vi "save_and_process_continious_image_data.vi"(0 "queue out":refnum<queue>, 1 "HDFvsTDMS":bool, 2 "Enable online recon":bool, 3 "Save":bool, 4 "Path for TDMS":path=path "C:/Users/MPI/Desktop", 5 "Subject metadata cluster":T2, 6 "Path":path=path "C:/Users/MPI/Desktop", 7 "System Information cluster":T1, 10 "OnlineReconPath":path) -> ()   [LabVIEW 2021]
uses:
  Human_Labview/global_variables.vi
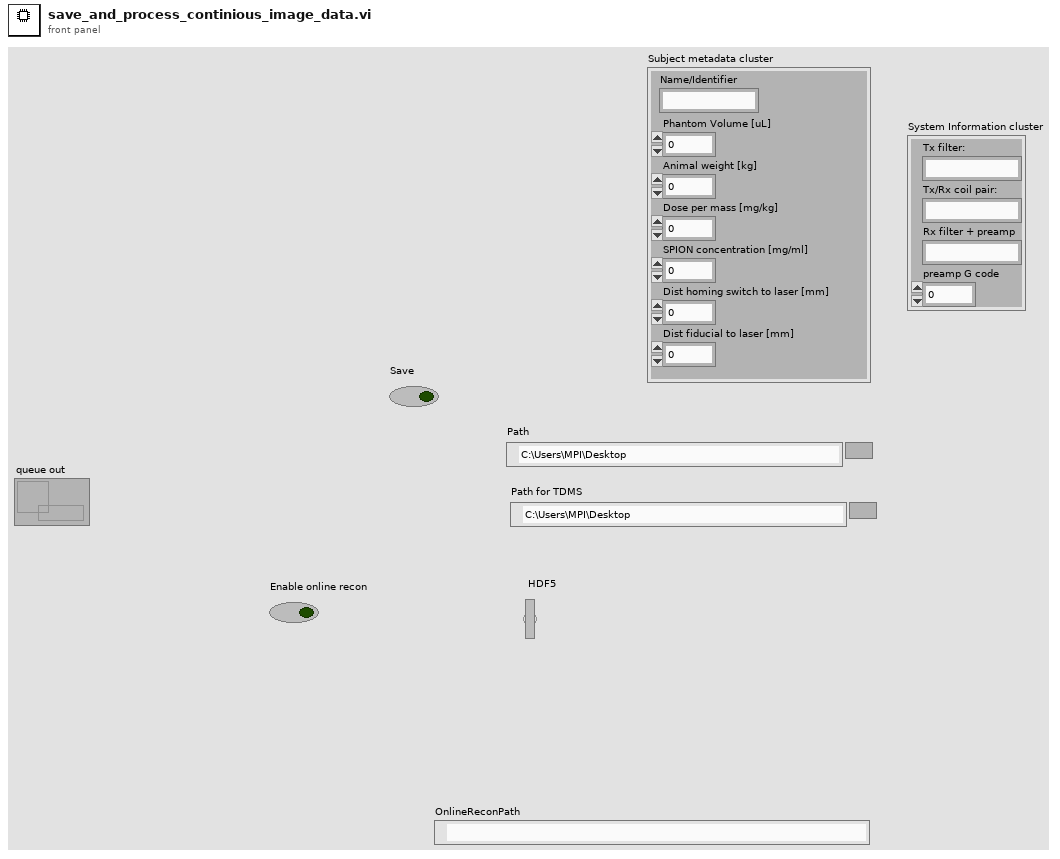
[diagram p1: front panel]
types:
  T1 = cluster{"Tx filter:":string, "Tx/Rx coil pair:":string, "Rx filter + preamp":string, "preamp G code":dbl}
  T2 = cluster{"Name/Identifier":string, "Phantom Volume [uL]":dbl, "Animal weight [kg]":dbl, "Dose per mass [mg/kg]":dbl, "SPION concentration [mg/ml]":dbl, "Dist homing switch to laser [mm]":dbl, "Dist fiducial to laser [mm]":dbl}
  T3 = cluster{"sample rate":dbl, "Transmit frequency":dbl, "Transmit amplitude":dbl, "sample rate digital out":dbl, "TX cycles":i32, "sample rate DAQ1":dbl, "Receive frequency":dbl, "Receive range":dbl, "TX harmonics":dbl[]}
  T4 = cluster{"Magnitude meas.":dbl[], "Phase meas.":dbl[], "Shift meas.":dbl[], "cw":bool, "projections per image":i32, "ramp-up readouts":i32, "current sense type":string, "Number of pulses per image":i32, "Rotation enabled":bool, "Rotary position":dbl[], "Baseline magnitude":dbl, "Baseline phase":dbl, "Wait readouts":i32, "Shift waveform type":string, "Shift enabled":bool, "Time domain data":dbl[], "Motor pulse duration":dbl, "Shift start":dbl, "Shift stop":dbl, "Notes":string, "Reconstructed image":picture, "Rotary encoder type":string, "Image start":timestamp, "Image stop":timestamp, "readouts per projection":i32, "Recon enabled":bool, "Bidirectional shift":bool, "Imager mode":string, "Shift delay":dbl, "Shift frequency":dbl, "Image time (calc)":dbl, "Initial encoder position":dbl, "Recon data":dbl[][], "Trigger line values":i32[], "Bed position":dbl, "Sample image":picture, "Patch amplitude":dbl, "Patch frequency":dbl, "Patch phase":dbl, "proj mag f2-f9":dbl[][], "proj phase f2-f9":dbl[][], "Tx waveform":dbl[], "Tx FFT mag":dbl[], "Tx FFT phase":dbl[], "Temps":dbl[]}
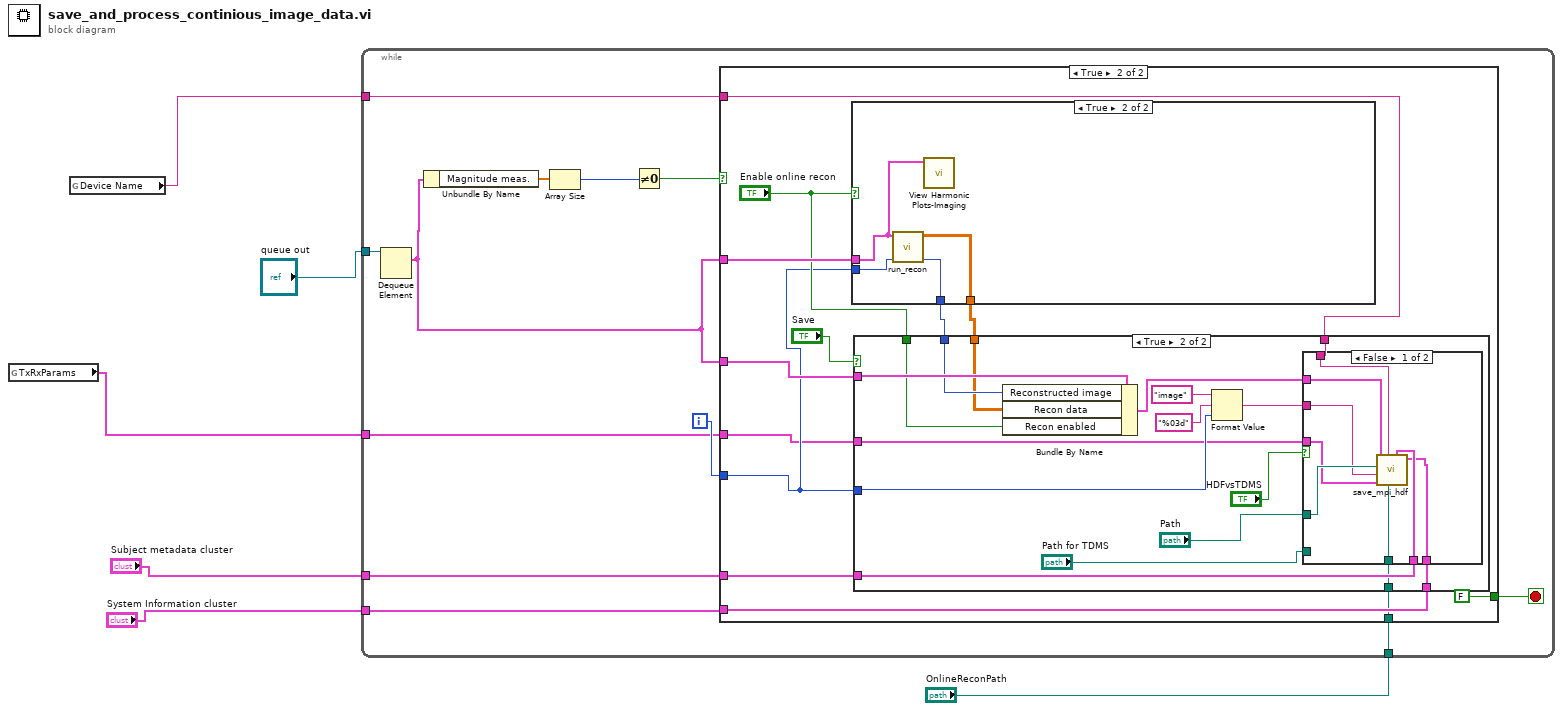
[diagram p0: block diagram]
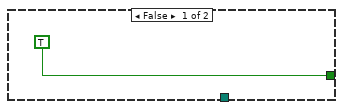
[diagram p2: hidden frame]
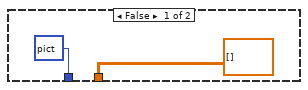
[diagram p3: hidden frame]
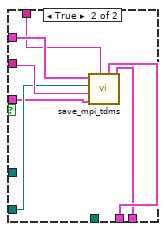
[diagram p5: hidden frame]
diagram:
  n1 = global read "global_variables.vi" "TxRxParams"() -> (w5:T3)
  n2 = global read "global_variables.vi" "Device Name"() -> (w4:tag)
  n3 = while {
    tunnel: "queue out" -> [w15]
    tunnel: w5 -> [w11]
    tunnel: w4 -> [w10]
    tunnel: "Subject metadata cluster" -> [w9]
    tunnel: "System Information cluster" -> [w8]
    tunnel: "OnlineReconPath" -> [w7]
    i -> [w13]
    stop <- w14 stop-if-true
    n4 = Dequeue Element(queue=w15) -> (element=w12:T4)  [unwired: 2 in, 3 out]
    n5 = Unbundle By Name(w12) -> ("Magnitude meas."=w18:dbl[])
    n6 = Array Size(array=w18) -> (size(s)=w17:i32)
    n7 = Not Equal To 0?(x=w17) -> (x != 0?=w16:bool)
    n8 = case shown="True" w16 {
      tunnel: [TRUE FALSE] -> w14
      tunnel: w13 -> [_ w25]
      tunnel: w12 -> [_ w31]
      tunnel: w12 -> [_ w30]
      tunnel: w11 -> [_ w24]
      tunnel: w10 -> [_ w23]
      tunnel: w9 -> [_ w22]
      tunnel: w8 -> [_ w21]
      tunnel: w7 -> [_ w20]
      frame False {
      }
      frame True {
        n9 = case shown="True" "Enable online recon" {
          tunnel: w31 -> [_ w36]
          tunnel: [picture data[5B] ("Reconstructed image") w38] -> w29
          tunnel: [dbl[][] [] ("Recon data") w35] -> w28
          tunnel: w25 -> [_ w37]
          frame False {
          }
          frame True {
            n10 = call "run_recon.vi"("image number"=w37, "Cluster in"=w36) -> ("reconstructed image"=w38:picture, "Recon data"=w35:dbl[][])  [unwired: 6 in, 2 out]
            n11 = call "View Harmonic Plots-Imaging.vi"("Cluster in"=w36) -> ()  [unwired: 11 in]
          }
        }
        n12 = case shown="True" "Save" {
          tunnel: w25 -> [_ w53]
          tunnel: w30 -> [_ w52]
          tunnel: w29 -> [_ w51]
          tunnel: w28 -> [_ w50]
          tunnel: "Enable online recon" -> [_ w49]
          tunnel: w24 -> [_ w43]
          tunnel: w23 -> [_ w42]
          tunnel: w22 -> [_ w41]
          tunnel: w21 -> [_ w40]
          tunnel: w20 -> [_ w39]
          frame False {
          }
          frame True {
            n13 = Bundle By Name(cluster=w52, "Reconstructed image"=w51, "Recon data"=w50, "Recon enabled"=w49) -> (w48:T4)
            n14 = Format Value(string ("")="image", format string="%03d", value (0)=w53) -> (output string=w46:string)
            n15 = case shown="False" "HDFvsTDMS" {
              tunnel: w48 -> [w61 w70]
              tunnel: "Path" -> [w63 _]
              tunnel: w46 -> [w62 w69]
              tunnel: "Path for TDMS" -> [_ w68]
              tunnel: w43 -> [w60 w67]
              tunnel: w42 -> [w59 w66]
              tunnel: w41 -> [w58 w65]
              tunnel: w40 -> [w57 w64]
              tunnel: w39 -> [w56 _]
              frame False {
                n16 = call "save_mpi_hdf.vi"("System Information cluster"=w57, "Subject metadata cluster"=w58, "OnlineReconPath"=w56, "Device Name"=w59, "TxRxParams"=w60, "image dataset"=w62, "Path"=w63, "Cluster in"=w61) -> ()  [unwired: 4 in]
              }
              frame True {
                n17 = call "save_mpi_tdms.vi"("System Information cluster"=w64, "Subject metadata cluster"=w65, "Device Name"=w66, "TxRxParams"=w67, "image dataset"=w69, "Path"=w68, "Cluster in"=w70) -> ()  [unwired: 5 in]
              }
            }
          }
        }
      }
    }
  }
